vi "DBL to String.vi"(11 "Numeric":dbl) -> (3 "String":string)   [LabVIEW 2016, in "SLL String.lvlib"]
uses:
  SLL String.lvlib
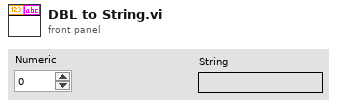
[diagram p1: front panel]
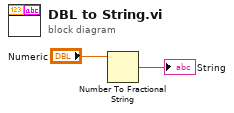
[diagram p0: block diagram]
diagram:
  n1 = Number To Fractional String(number="Numeric") -> (F-format string=→"String":string)  [unwired: 3 in]
